vi "SC10_open_shutter.vi"() -> ()   [LabVIEW 2010]
panel:
  in  "time (ms)":i32
  out "substring":string
  in  "VISA resource name":refnum<visa-resource-name>
  out "VISA resource name out":refnum<visa-resource-name>
  out "read buffer":string
  out "return count 2":u32
  out "return count":u32
  out "error out":errorcluster
  in  "error in (no error)":errorcluster
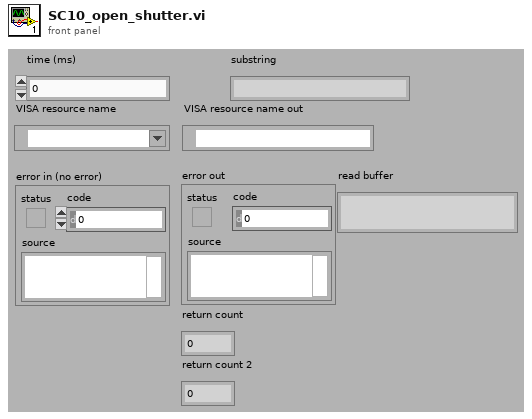
[diagram p1: front panel]
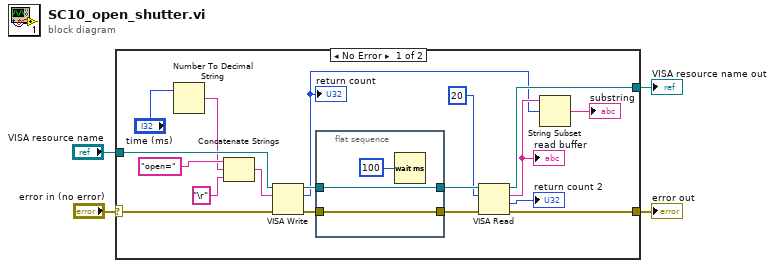
[diagram p0: block diagram]
diagram:
  n1 = case shown="No Error" "error in (no error)" {
    selector: "error in (no error)" -> [w18 w26]
    tunnel: [w17 w26] -> w3
    tunnel: [w14 w27] -> w2
    tunnel: "VISA resource name" -> [w13 w27]
    frame No Error {
      n2 = Number To Decimal String(number="time (ms)") -> (decimal integer string=w6:string)  [unwired: 1 in]
      n3 = Concatenate Strings("open=" ("string"), w6, "\r" ("write buffer")) -> (w7:string)
      n4 = VISA Write(VISA resource name=w13, write buffer=w7, error in (no error)=w18) -> (VISA resource name out=w22:refnum<visa-resource-name>, return count=w10:u32, error out=w20:errorcluster)
      "return count" <- w10
      n5 = flat-sequence {
        tunnel: w22 -> [w24]
        tunnel: [w24] -> w21
        tunnel: w20 -> [w23]
        tunnel: [w23] -> w19
        frame #0 {
          n6 = Wait (ms)(milliseconds to wait=u32 100) -> ()  [unwired: 1 out]
        }
      }
      n7 = VISA Read(VISA resource name=w21, byte count=u32 20, error in (no error)=w19) -> (VISA resource name out=w14:refnum<visa-resource-name>, read buffer=w12:string, return count=→"return count 2":u32, error out=w17:errorcluster)
      "read buffer" <- w12
      n8 = String Subset(string=w12, offset (0)=w10) -> (substring=→"substring":string)  [unwired: 1 in]
    }
    frame Error {
    }
  }
  "error out" <- w3
  "VISA resource name out" <- w2
